vi "bh3_acc100mg_waveform_format.vi"(11 "Acc 100mg Waveform Packet":u8[](array[numeric]) format="%02x") -> (2 "acc (G)":dbl[][](array[numeric]), 3 "counter":u8, 4 "milliseconds":u32, 5 "month":u8, 6 "day":u8, 7 "year":u16)   [LabVIEW 2013]
panel:
  out "output array":bool[][](array[boolean])
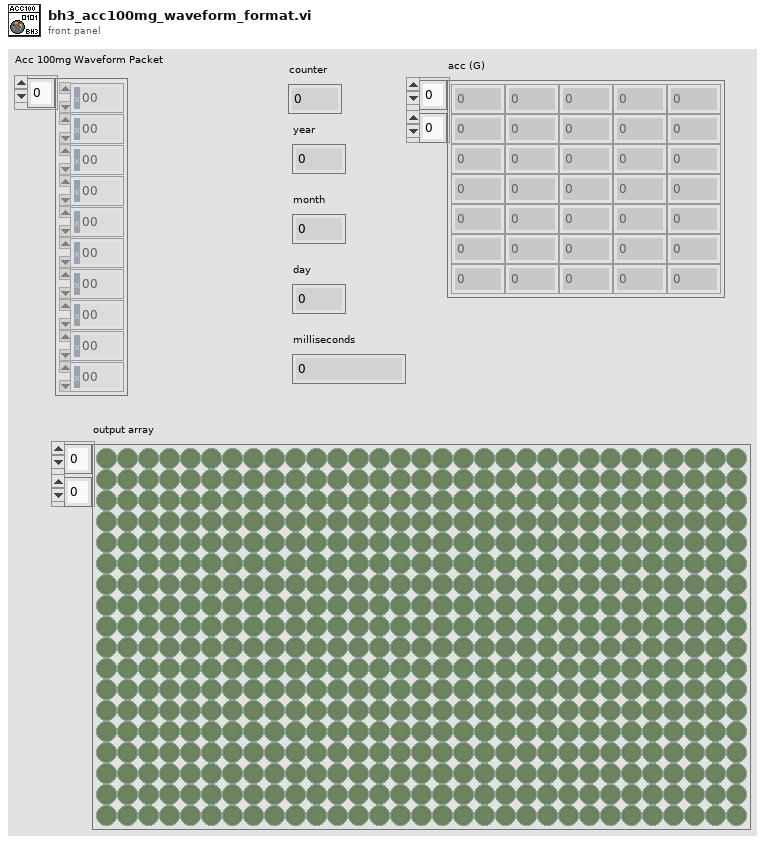
[diagram p1: front panel]
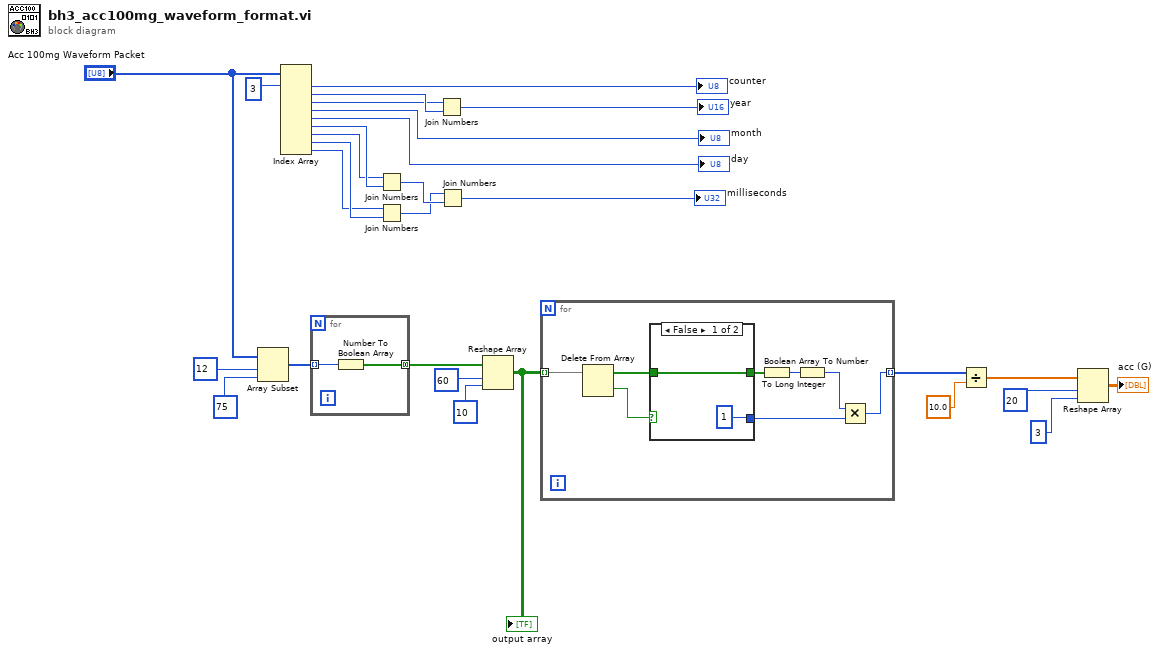
[diagram p0: block diagram]
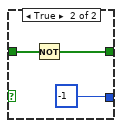
[diagram p2: hidden frame]
diagram:
  n1 = Array Subset(array="Acc 100mg Waveform Packet", index=12, length=75 ("index")) -> (w7:u8[])
  n2 = Index Array(array="Acc 100mg Waveform Packet", index #1=3 ("index")) -> (element #1=→"counter":u8, element #2=w28:u8, element #3=w27:u8, element #4=→"month":u8, element #5=→"day":u8, element #6=w21:u8, element #7=w20:u8, element #8=w17:u8, element #9=w16:u8)  [unwired: 8 in]
  n3 = for {
    tunnel: w7 -> [w30] mode=indexing
    tunnel: [w29] -> w11 mode=concatenating
    n4 = Number To Boolean Array(number=w30) -> (Boolean array=w29:bool[])
  }
  n5 = Join Numbers(hi=w20, lo=w21) -> ((hi.lo)=w19:u16)
  n6 = Join Numbers(hi=w16, lo=w17) -> ((hi.lo)=w18:u16)
  n7 = Join Numbers(hi=w27, lo=w28) -> ((hi.lo)=→"year":u16)
  n8 = Join Numbers(hi=w18, lo=w19) -> ((hi.lo)=→"milliseconds":u32)
  n9 = Reshape Array(w11, 60 ("dimension size"), 10 ("dimension size")) -> (w8:bool[][])
  "output array" <- w8
  n10 = for {
    tunnel: w8 -> [w38] mode=indexing
    tunnel: [w32] -> w5 mode=indexing
    n11 = Delete From Array(array=w38) -> (deleted portion=w36:bool, array with subset deleted=w34:bool[])  [unwired: 2 in]
    n12 = case shown="False" w36 {
      tunnel: [w40 w43] -> w35
      tunnel: w34 -> [w40 w42]
      tunnel: [1 ("dimension size") -1 ("dimension size")] -> w31
      frame False {
      }
      frame True {
        n13 = Not(x=w42) -> (.not. x?=w43:bool[])
      }
    }
    n14 = Boolean Array To Number(Boolean array=w35) -> (number=w37:u32)
    n15 = To Long Integer(number=w37) -> (32bit integer=w33:i32)
    n16 = Multiply(x=w33, y=w31) -> (x*y=w32:i32)
  }
  n17 = Divide(x=w5, y=10.0) -> (x/y=w4:dbl[])
  n18 = Reshape Array(w4, 20 ("dimension size"), 3 ("dimension size")) -> (→"acc (G)":dbl[][])
